vi "OpenConnection.vi"(0 "STOMP in":refnum<class "STOMP.lvclass">, 1 "address":string="localhost", 2 "port":u16=61613, 4 "timeout ms (60000)":i32=10000, 5 "error in (no error)":errorcluster) -> (14 "STOMP out":refnum<class "STOMP.lvclass">, 19 "error out":errorcluster)   [LabVIEW 2017, in "STOMP.lvclass"]
uses:
  STOMP.lvclass
  STOMP.lvclass/STOMP.ctl
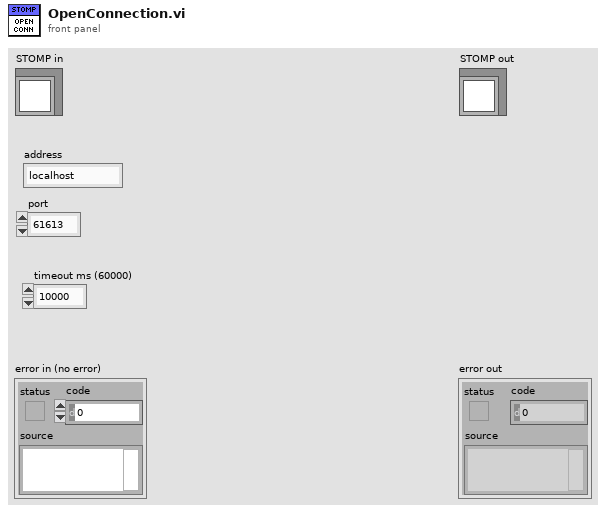
[diagram p1: front panel]
types:
  T1 = typedef "LabVIEW STOMP.lvlib/STOMP.lvclass/ObjectAttributes.ctl" = cluster{"address":string, "port":u16, "ConnectionRef":refnum<k5>, "messageQueue":refnum<queue>, "receiptQueue":refnum<queue>, "errorQueue":refnum<queue>, "sendQueue":refnum<queue>, "currentReceiptNumber":u64, "currentSubscriptionId":u64, "closeConnection":bool, "activeSubscriptions":T2[]}
  T2 = typedef "Type_ActiveSubscription.ctl" = cluster{"id":u64, "receipt":bool, "Destination":string, "ack":T3, "headers":T4[]}
  T3 = typedef "Type_AckHeader.ctl" = enum16{"auto", "client", "client-individual"}
  T4 = typedef "LabVIEW STOMP.lvlib/STOMP.lvclass/Type_FrameHeader.ctl" = cluster{"Header":string, "Value":string}
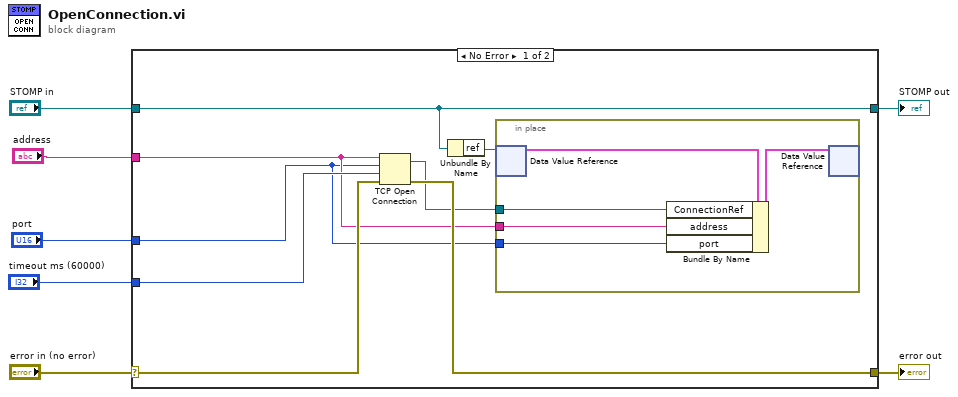
[diagram p0: block diagram]
diagram:
  n1 = case shown="No Error" "error in (no error)" {
    selector: "error in (no error)" -> [w14 w22]
    tunnel: [w13 w22] -> w6
    tunnel: [w8 w21] -> w4
    tunnel: "STOMP in" -> [w8 w21]
    tunnel: "timeout ms (60000)" -> [w15 _]
    tunnel: "port" -> [w10 _]
    tunnel: "address" -> [w11 _]
    frame No Error {
      n2 = TCP Open Connection(address=w11, remote port or service name=w10, timeout ms (60000)=w15, error in (no error)=w14) -> (connection ID=w9:refnum<k5>, error out=w13:errorcluster)  [unwired: 1 in]
      n3 = Unbundle By Name(w8) -> ("ref"=w12:refnum<data-value>)
      n4 = in-place {
        in-place-border: w11 -> [w18]
        in-place-border: w10 -> [w17]
        in-place-border: w9 -> [w16]
        n5 = in-place-dvr #1(w12) -> (w20:T1)  [unwired: 1 out]
        n6 = Bundle By Name(cluster=w20, "ConnectionRef"=w16, "address"=w18, "port"=w17) -> (w19:T1)
        n7 = in-place-dvr #1(w19) -> ()  [unwired: 2 out]
      }
    }
    frame Error {
    }
  }
  "error out" <- w6
  "STOMP out" <- w4
